vi "test_LocationFGV_GetLocationTwice_LocationResolvedOnce.vi"(8 "error in":errorcluster) -> (0 "error out":errorcluster, 2 "result":string, 3 "pass":bool)   [LabVIEW 2020, in "MeasurementServerTests.lvlib" / "gRPC Utilities Tests.lvlib"]
uses:
  gRPC Utilities Tests.lvlib
  Fake Location Action.ctl
  Runtime/MeasurementLink Discovery/TypeDefs/Service Location FGV Action.ctl
  Runtime/MeasurementLink Discovery/MeasurementLink Discovery.lvlib
  Runtime/MeasurementLink Discovery Client/RPC Messages/ni_measurementlink_discovery_v1_ResolveServiceRequest.ctl
  Runtime/MeasurementLink Discovery Client/MeasurementLink Discovery Client.lvlib
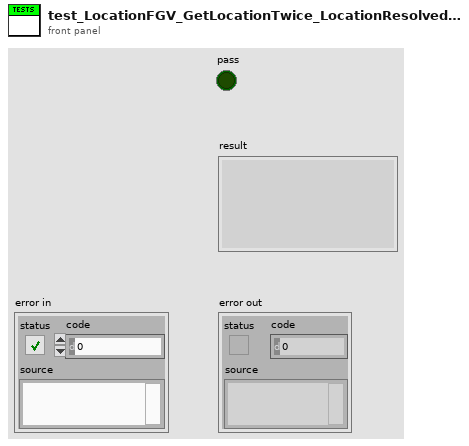
[diagram p1: front panel]
types:
  T1 = typedef "MeasurementLink Discovery Client.lvlib/ni_measurementlink_discovery_v1_ResolveServiceRequest.ctl" = cluster{"provided_interface":string, "service_class":string}
  T2 = typedef "MeasurementLink Discovery.lvlib/Service Location FGV Action.ctl" = enum16{"Get Service Location", "Reresolve Service Location"}
  T3 = typedef "MeasurementServerTests.lvlib/gRPC Utilities Tests.lvlib/Fake Location Action.ctl" = enum16{"Generate New Location", "Reset", "Error on Next Call"}
  T4 = typedef "MeasurementLink Discovery Client.lvlib/ni_measurementlink_discovery_v1_ServiceLocation.ctl" = cluster{"location":string, "insecure_port":string, "ssl_authenticated_port":string}
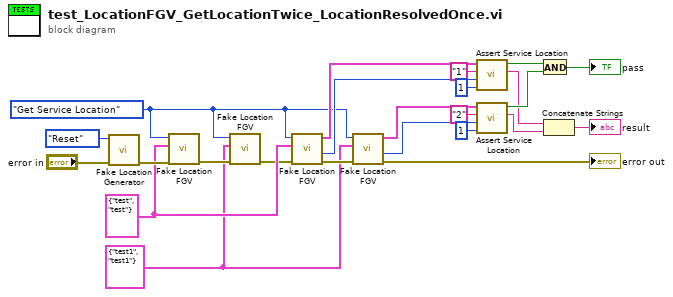
[diagram p0: block diagram]
diagram:
  w12 = T1 {"provided_interface"="test1", "service_class"="test1"} ("resolve service request")
  w21 = T1 {"provided_interface"="test", "service_class"="test"} ("resolve service request")
  w13 = Service_Location_FGV_Action."Get Service Location" ("action")
  n1 = call "Fake Location Generator.vi"("error in"="error in", "action"=Fake_Location_Action."Reset") -> ("error out"=w23:errorcluster)  [unwired: 8 in, 1 out]
  n2 = call "Fake Location FGV.vi"("error in"=w23, "resolve service request"=w21, "action"=w13) -> ("error out"=w16:errorcluster)  [unwired: 6 in, 2 out]
  n3 = call "Fake Location FGV.vi"("error in"=w16, "resolve service request"=w12, "action"=w13) -> ("error out"=w15:errorcluster)  [unwired: 6 in, 2 out]
  n4 = call "Fake Location FGV.vi"("error in"=w15, "resolve service request"=w21, "action"=w13) -> ("error out"=w14:errorcluster, "unique id out"=w18:u64, "service location"=w20:T4)  [unwired: 6 in]
  n5 = call "Fake Location FGV.vi"("error in"=w14, "resolve service request"=w12, "action"=w13) -> ("error out"=→"error out":errorcluster, "unique id out"=w7:u64, "service location"=w8:T4)  [unwired: 6 in]
  n6 = call "Assert Service Location.vi"("expected unique id"=u64 1, "actual unique id"=w18, "expected service location port"="1", "actual service location"=w20) -> ("result"=w3:string, "pass"=w17:bool)  [unwired: 6 in]
  n7 = call "Assert Service Location.vi"("expected unique id"=u64 1, "actual unique id"=w7, "expected service location port"="2", "actual service location"=w8) -> ("result"=w2:string, "pass"=w4:bool)  [unwired: 6 in]
  n8 = And(x=w17, y=w4) -> (x .and. y?=→"pass":bool)
  n9 = Concatenate Strings(w3, w2) -> (→"result":string)
